vi "Image Threshold.vi"() -> ()   [LabVIEW 2014]
doc: "This example illustrates different thresholding algorithms. Local thresholding calculates local statistics for each pixel in an image. Based on the calculation result, the algorithm categorizes the pixel as part of a particle or the background. Automatic thresholding uses the histogram of an image to compute a single threshold value for the entire image. Manual thresholding uses a specified range of values to compute a threshold value for the image. Refer to the NI Vision Concepts Manual for more information about thresholding algorithms."
uses:
  <vilib>/vision/NI_Vision_Development_Module.lvlib
panel:
  in  "Threshold Type":enum32{"Local", "Automatic", "Manual"}(tab)
  in  "Local":T1={"Object Type"=1, "Method"=1, "Niblack Deviation Factor"=1.0, "Window"={"Width"=160, "Height"=160}} {"Niblack Deviation Factor" min=0.0 max=1.0 format="%.2f"; "Method" items=["Niblack", "Background Correction"]; "Object Type" items=["Bright Objects", "Dark Objects"]}
  in  "Automatic":cluster{"Object Type":u32, "Method":i32}={"Object Type"=1, "Method"=0} {"Method" items=["clustering", "entropy", "metric", "moments", "inter-class variance"]; "Object Type" items=["Bright Objects", "Dark Objects"]}
  in  "Manual":cluster{sgl, sgl}(slide)={0.0, 150.0} caption="Threshold Range" scale=0.0..255.0
  out "Original":T2(plugin-control)
  in  "Stop":bool
  out "Threshold Image":T2(plugin-control)
  # "Overview: Demonstrates how to use different Threshold functions with an unevenly lit LCD display.\nRequirements: Vision Development Software.\nInstructions:\n1. Run the VI.\n2. Click on the different Threshold algorithm tabs to see how each algorithm works. The local threshold is the most robust algorithm when there are lighting variations in the image."
  # "Minimum"
  # "Maximum"
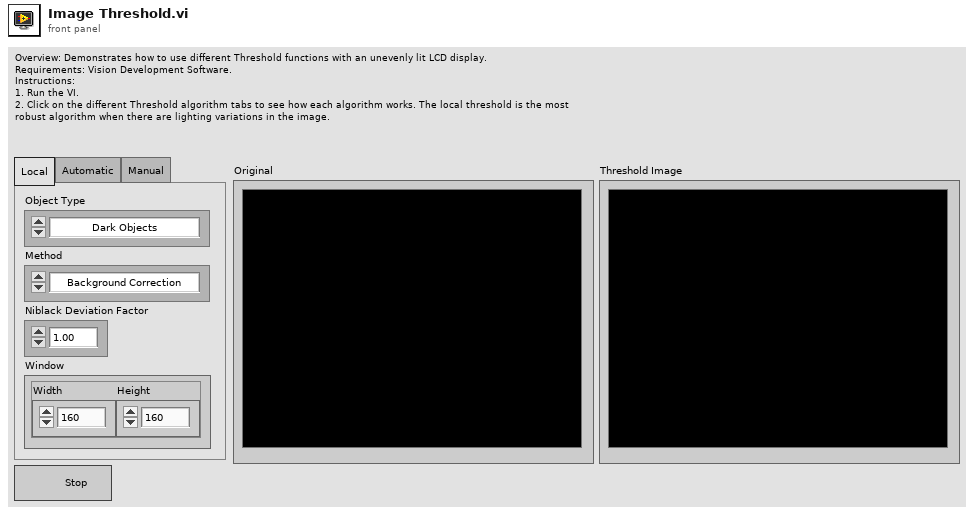
[diagram p1: front panel]
types:
  T1 = cluster{"Object Type":u32, "Method":u32, "Niblack Deviation Factor":dbl, "Window":cluster{"Width":i32, "Height":i32}}
  T2 = typedef "IMAQ Image.ctl" = refnum<image>
  T3 = cluster{"Threshold Type":enum32{"Local", "Automatic", "Manual"}, "Local":cluster{"Object Type":u32, "Method":u32, "Niblack Deviation Factor":dbl, "Window":cluster{"Width":i32, "Height":i32}}, "Automatic":cluster{"Object Type":u32, "Method":i32}, "Manual":cluster{sgl, sgl}}
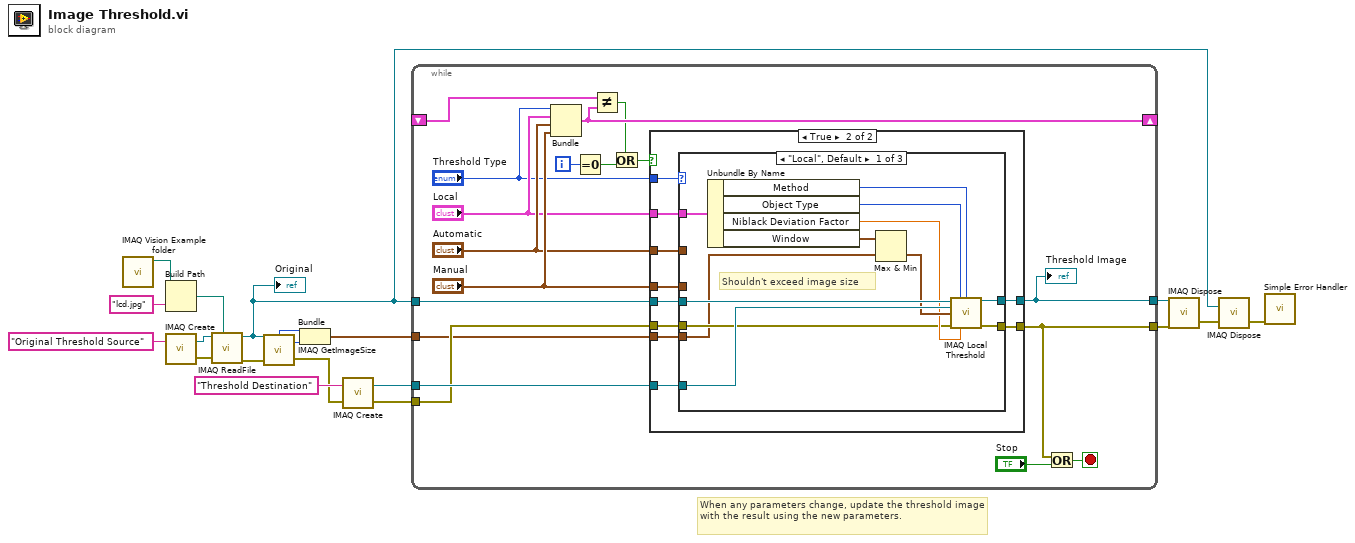
[diagram p0: block diagram]
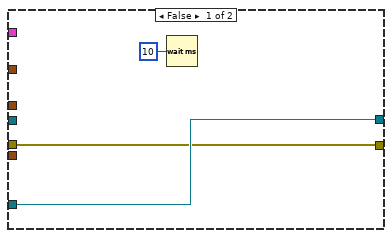
[diagram p2: hidden frame]
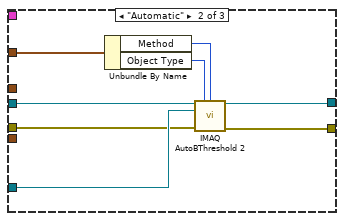
[diagram p3: hidden frame]
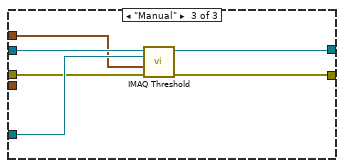
[diagram p4: hidden frame]
diagram:
  # "When any parameters change, update the threshold image with the result using the new parameters."
  n1 = call "IMAQ Vision Example folder.vi"() -> ("Example Image Path"=w15:path)  [unwired: 11 in]
  n2 = Build Path(base path=w15, name or relative path="lcd.jpg") -> (appended path=w13:path)
  n3 = call "IMAQ Create"("Image Name"="Original Threshold Source") -> ("New Image"=w12:T2, "error out"=w11:errorcluster)  [unwired: 4 in]
  n4 = call "IMAQ ReadFile"("File Path"=w13, "error in (no error)"=w11, "Image"=w12) -> ("error out"=w14:errorcluster, "Image Out"=w3:T2)  [unwired: 4 in, 3 out]
  "Original" <- w3
  n5 = call "IMAQ GetImageSize"("Image"=w3, "error in (no error)"=w14) -> ("Y Resolution"=w8:i32, "X Resolution"=w9:i32, "error out"=w10:errorcluster)  [unwired: 2 in]
  n6 = Bundle("X Resolution"=w9, "Y Resolution"=w8) -> (w1:cluster{"X Resolution":i32, "Y Resolution":i32})  [unwired: 1 in]
  n7 = call "IMAQ Create"("Image Name"="Threshold Destination", "error in (no error)"=w10) -> ("New Image"=w19:T2, "error out"=w7:errorcluster)  [unwired: 3 in]
  n8 = while {
    tunnel: w3 -> [w37]
    tunnel: w19 -> [w36]
    tunnel: w7 -> [w27]
    shift-right: [w31] -> _
    shift-left: _ -> [w30]
    tunnel: [w21] -> w5
    tunnel: [w28] -> w6
    tunnel: w1 -> [w26]
    i -> [w25]
    stop <- w29 stop-if-true
    n9 = Bundle("Threshold Type"="Threshold Type", "Local"="Local", "Automatic"="Automatic", "Manual"="Manual") -> (w31:T3)  [unwired: 1 in]
    n10 = Equal To 0?(x=w25) -> (x = 0?=w24:bool)
    n11 = Not Equal?(x=w30, y=w31) -> (x != y?=w22:bool)
    n12 = Or(x=w22, y=w24) -> (x .or. y?=w23:bool)
    n13 = case shown="True" w23 {
      tunnel: w37 -> [_ w50]
      tunnel: w36 -> [w40 w49]
      tunnel: [w40 w48] -> w28
      tunnel: "Manual" -> [_ w47]
      tunnel: "Automatic" -> [_ w46]
      tunnel: "Local" -> [_ w45]
      tunnel: "Threshold Type" -> [_ w44]
      tunnel: [w38 w43] -> w21
      tunnel: w27 -> [w38 w42]
      tunnel: w26 -> [_ w41]
      frame False {
        n14 = Wait (ms)(milliseconds to wait=u32 10) -> ()  [unwired: 1 out]
      }
      frame True {
        n15 = case shown="\"Local\", Default" w44 {
          tunnel: w50 -> [w62 w70 w76]
          tunnel: w49 -> [w61 w69 w75]
          tunnel: [w60 w68 w74] -> w48
          tunnel: w45 -> [w59 _ _]
          tunnel: w46 -> [_ w67 _]
          tunnel: [w53 w66 w72] -> w43
          tunnel: w47 -> [_ _ w73]
          tunnel: w42 -> [w52 w63 w71]
          tunnel: w41 -> [w51 _ _]
          frame "Local", Default {
            # "Shouldn't exceed image size"
            n16 = Unbundle By Name(w59) -> ("Method"=w57:u32, "Object Type"=w56:u32, "Niblack Deviation Factor"=w55:dbl, "Window"=w54:cluster{"Width":i32, "Height":i32})
            n17 = Max & Min(x=w54, y=w51) -> (min(x,y)=w58:cluster{i32, i32})  [unwired: 1 out]
            n18 = call "IMAQ Local Threshold"("Image Src"=w62, "Look For (Bright Objects)"=w56, "Method (Niblack)"=w57, "Image Dst"=w61, "Window Size (32x32)"=w58, "error in (no error)"=w52, "Niblack Deviation Factor (0.2)"=w55) -> ("Image Dst Out"=w60:T2, "error out"=w53:errorcluster)  [unwired: 7 in]
          }
          frame "Automatic" {
            n19 = Unbundle By Name(w67) -> ("Method"=w65:i32, "Object Type"=w64:u32)
            n20 = call "IMAQ AutoBThreshold 2"("Image Src"=w70, "Look For (Bright Objects)"=w64, "Method (clustering)"=w65, "Image Dst"=w69, "error in (no error)"=w63) -> ("Image Dst Out"=w68:T2, "error out"=w66:errorcluster)  [unwired: 8 in, 1 out]
          }
          frame "Manual" {
            n21 = call "IMAQ Threshold"("error in (no error)"=w71, "Range"=w73, "Image Dst"=w75, "Image Src"=w76) -> ("error out"=w72:errorcluster, "Image Dst Out"=w74:T2)  [unwired: 6 in]
          }
        }
      }
    }
    "Threshold Image" <- w28
    n22 = Or(x=w21, y="Stop") -> (x .or. y?=w29:bool)
  }
  n23 = call "IMAQ Dispose"("Image"=w6, "error in (no error)"=w5) -> ("error out"=w4:errorcluster)  [unwired: 4 in]
  n24 = call "IMAQ Dispose"("Image"=w3, "error in (no error)"=w4) -> ("error out"=w2:errorcluster)  [unwired: 4 in]
  n25 = call <vilib>:"Simple Error Handler.vi"("error in (no error)"=w2) -> ()  [unwired: 4 in, 5 out]
